vi "TDMS_DBL_Array to file.vi"(5 "Interval":T1=enum."Daily", 6 "channel name(s) in":string[](array[string])=["Time", "Distance"], 7 "group name in (Untitled)":string="SonarAlt", 8 "error in (no error)":errorcluster, 9 "Data":dbl[](array[numeric]), 10 "FilePrefix":string, 11 "Base path":path) -> (0 "error out":errorcluster, 3 "sonic file out":refnum<k34>)   [LabVIEW 2025]
uses:
  Enum_FileNewInterval.ctl
  4eaa4cfa-5103-44e1-8cfa-05a335443445.vi
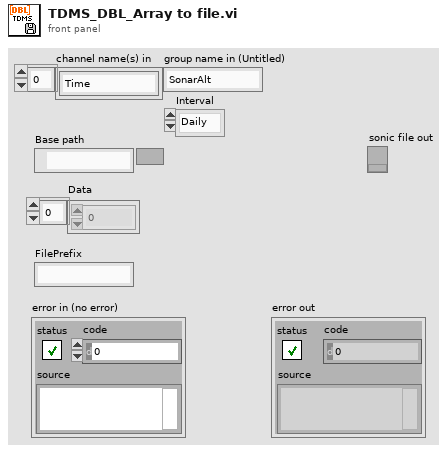
[diagram p1: front panel]
types:
  T1 = typedef "Enum_FileNewInterval.ctl" = enum16{"2 Min", "10 Min", "Hourly", "Daily", "Weekly", "Monthly"}
  T2 = enum16{"open", "open or create", "create or replace", "create", "open (read-only)"}
  T3 = typedef "LVDateTimeRec.ctl" = cluster{"fractional second":dbl, "second":i32, "minute":i32, "hour":i32, "day of month":i32, "month":i32, "year":i32, "day of week":i32, "day of year":i32, "DST":i32}
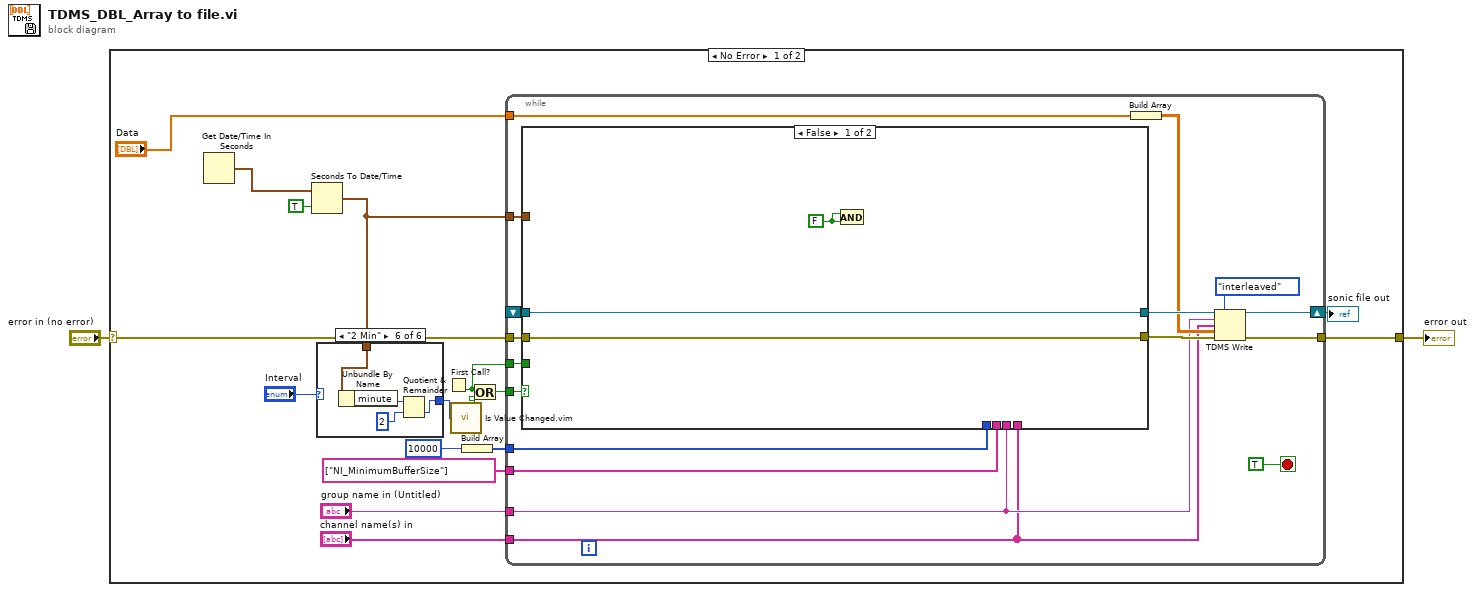
[diagram p0: block diagram]
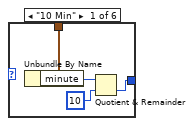
[diagram p2: hidden frame]
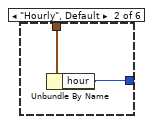
[diagram p3: hidden frame]
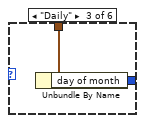
[diagram p4: hidden frame]
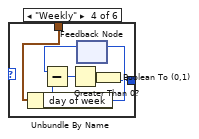
[diagram p5: hidden frame]
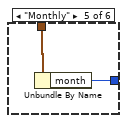
[diagram p6: hidden frame]
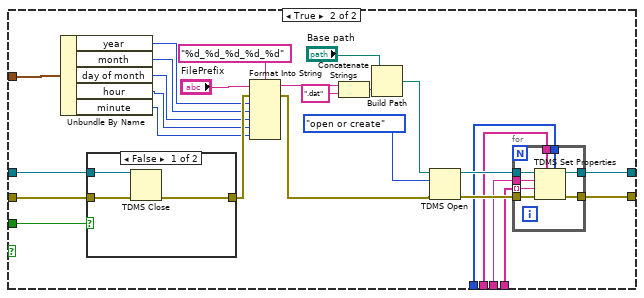
[diagram p7: hidden frame]
diagram:
  n1 = case shown="No Error" "error in (no error)" {
    selector: "error in (no error)" -> [w15 w99]
    tunnel: [w17 w99] -> w2
    frame No Error {
      n2 = Get Date/Time In Seconds() -> (seconds since 1Jan1904=w6:timestamp)
      n3 = Seconds To Date/Time(time stamp (now)=w6, to UTC (F)=TRUE) -> (date time rec=w5:T3)
      n4 = case shown="\"2 Min\"" "Interval" {
        tunnel: w5 -> [w23 w25 w27 w33 w35 w37]
        tunnel: [w20 w24 w26 w28 w34 w36] -> w4
        frame "10 Min" {
          n5 = Unbundle By Name(w23) -> ("minute"=w22:i32)
          n6 = Quotient & Remainder(x=w22, y=10) -> (floor(x/y)=w20:i32)  [unwired: 1 out]
        }
        frame "Hourly", Default {
          n7 = Unbundle By Name(w25) -> ("hour"=w24:i32)
        }
        frame "Daily" {
          n8 = Unbundle By Name(w27) -> ("day of month"=w26:i32)
        }
        frame "Weekly" {
          n9 = Unbundle By Name(w33) -> ("day of week"=w31:i32)
          n10 = feedback-in #1(w31) -> ()
          n11 = feedback #1() -> (w32:i32)  [unwired: 1 in]
          n12 = Subtract(x=w32, y=w31) -> (x-y=w30:i32)
          n13 = Greater Than 0?(x=w30) -> (x > 0?=w29:bool)
          n14 = Boolean To (0,1)(Boolean=w29) -> (0, 1=w28:i16)
        }
        frame "Monthly" {
          n15 = Unbundle By Name(w35) -> ("month"=w34:i32)
        }
        frame "2 Min" {
          n16 = Unbundle By Name(w37) -> ("minute"=w39:i32)
          n17 = Quotient & Remainder(x=w39, y=2) -> (floor(x/y)=w36:i32)  [unwired: 1 out]
        }
      }
      n18 = First Call?() -> (First Call?: T/F=w18:bool)
      n19 = call "Is Value Changed.vim"("value"=w4) -> ("changed or first call?"=w3:bool)
      n20 = Build Array(10000) -> (w9:i32[])
      n21 = Or(x=w18, y=w3) -> (x .or. y?=w19:bool)
      n22 = while {
        tunnel: w19 -> [w56]
        shift-right: [w47] -> w16
        shift-left: _ -> [w55]
        tunnel: w18 -> [w54]
        tunnel: "Data" -> [w51]
        tunnel: [w46] -> w17
        tunnel: w15 -> [w53]
        tunnel: w5 -> [w50]
        tunnel: "channel name(s) in" -> [w40]
        tunnel: "group name in (Untitled)" -> [w41]
        tunnel: w9 -> [w43]
        tunnel: string[] ["NI_MinimumBufferSize"] ("Channel Names") -> [w42]
        stop <- TRUE stop-if-true
        n23 = case shown="False" w56 {
          tunnel: [w59 w65] -> w49
          tunnel: w55 -> [w59 w78]
          tunnel: w54 -> [_ w79]
          tunnel: [w58 w64] -> w48
          tunnel: w53 -> [w58 w77]
          tunnel: w50 -> [_ w68]
          tunnel: w43 -> [_ w63]
          tunnel: w42 -> [_ w62]
          tunnel: w41 -> [_ w61]
          tunnel: w40 -> [_ w60]
          frame False {
            w57 = FALSE ("y")
            n24 = And(x=w57, y=w57) -> ()  [unwired: 1 out]
          }
          frame True {
            n25 = Unbundle By Name(w68) -> ("year"=w76:i32, "month"=w75:i32, "day of month"=w74:i32, "hour"=w71:i32, "minute"=w70:i32)
            n26 = case shown="False" w79 {
              tunnel: w78 -> [w97 _]
              tunnel: [w96 w98] -> w86
              tunnel: w77 -> [w95 w98]
              frame False {
                n27 = TDMS Close(8:w95, 11:w97) -> (0:w96:errorcluster)  [unwired: 1 out]
              }
              frame True {
              }
            }
            n28 = Format Into String(format string="%d_%d_%d_%d_%d", initial string="FilePrefix", error in=w86, w76, w75, w74, w71, w70) -> (resulting string=w85:string, error out=w69:errorcluster)
            n29 = Concatenate Strings(w85, ".dat" ("string")) -> (w82:string)
            n30 = Build Path(base path="Base path", name or relative path=w82) -> (appended path=w81:path)
            n31 = TDMS Open(8:w69, 10:T2."open or create" ("operation (0:open)"), 11:w81) -> (0:w67:errorcluster, 3:w66:refnum<k34>)  [unwired: 4 in]
            n32 = for {
              tunnel: w66 -> [w94]
              tunnel: [w93] -> w65
              tunnel: w67 -> [w92]
              tunnel: [w91] -> w64
              tunnel: w62 -> [w90]
              tunnel: w63 -> [w89]
              tunnel: w61 -> [w88]
              tunnel: w60 -> [w87] mode=indexing
              n33 = TDMS Set Properties(5:w89, 7:w90, 8:w92, 9:w87, 10:w88, 11:w94) -> (0:w91:errorcluster, 3:w93:refnum<k34>)  [unwired: 2 out]
            }
          }
        }
        n34 = Build Array(w51) -> (w45:dbl[][])
        n35 = TDMS Write(0:w49, 1:enum16{"decimated", "interleaved"}."interleaved" ("data layout (0:decimated)"), 5:w41, 7:w40, 9:w45, 11:w48) -> (4:w47:refnum<k34>, 15:w46:errorcluster)  [unwired: 2 out]
      }
      "sonic file out" <- w16
    }
    frame Error {
    }
  }
  "error out" <- w2
